vi "Initialize.vi"(8 "error in":errorcluster, 11 "Plugin in":refnum<class "Sequencer with Output Values.lvclass">) -> (0 "error out":errorcluster, 3 "Plugin out":refnum<class "Sequencer with Output Values.lvclass">)   [LabVIEW 2024, in "Sequencer with Output Values.lvlib" / "Sequencer with Output Values.lvclass"]
uses:
  Sequencer with Output Values.lvclass
  C:/Program Files/National Instruments/LabVIEW 2024/vi.lib/FlexLogger/SDK/PluginSDK.lvlibp/PEFClasses/SDK/Plugin/Plugin.lvclass
  <vilib>/FlexLogger/SDK/PluginSDK.lvlibp/PEFClasses/SDK/Processing Element/Timing Parameters.ctl
  <vilib>/FlexLogger/SDK/PluginSDK.lvlibp/PEFClasses/SDK/Processing Element/Timing Method.ctl
  Params.ctl
  Step Settings.ctl
  Helper VIs/Cust UI.ctl
  Sequencer with Output Values.lvclass/Sequencer with Output Values.ctl
  <vilib>/FlexLogger/SDK/PluginSDK.lvlibp/PEFClasses/SDK/Producer Channel/Producer Channel.lvclass
  C:/Program Files/National Instruments/LabVIEW 2024/vi.lib/FlexLogger/SDK/PluginSDK.lvlibp/PEFClasses/SDK/Channel/Channel.lvclass
  Global Strings.vi
  <vilib>/FlexLogger/SDK/PluginSDK.lvlibp/PEFClasses/SDK/Plugin/ParameterAccess/Write Command.vi
  <vilib>/FlexLogger/SDK/PluginSDK.lvlibp/PEFClasses/SDK/Plugin/ParameterAccess/Read String.vi
  <vilib>/FlexLogger/SDK/PluginSDK.lvlibp/PEFClasses/SDK/Plugin/ParameterAccess/Write String.vi
  Settings UI.vi
  <vilib>/FlexLogger/SDK/PluginSDK.lvlibp/PEFClasses/SDK/Producer Channel/Create Producer Channel.vi
  <vilib>/FlexLogger/SDK/PluginSDK.lvlibp/PEFClasses/SDK/Plugin/Plugin.lvclass
  <vilib>/FlexLogger/SDK/PluginSDK.lvlibp/PEFClasses/SDK/Processing Element/Processing Element.lvclass
  <vilib>/FlexLogger/SDK/PluginSDK.lvlibp
  C:/Program Files/National Instruments/LabVIEW 2024/vi.lib/FlexLogger/SDK/PluginSDK.lvlibp/PEFClasses/SDK/Processing Element/Processing Element.lvclass
  C:/dev/niflexlogger-plugins/plugins/Sequencer with Output Values/source/Sequencer with Output Values/Sequencer with Output Values.lvclass
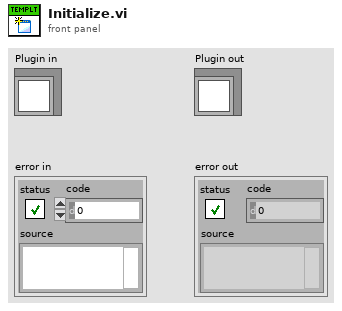
[diagram p1: front panel]
types:
  T1 = typedef "Sequencer with Output Values.lvlib/Sequencer with Output Values.lvclass/Cust UI.ctl" = refnum<vi>
  T2 = typedef "Sequencer with Output Values.lvlib/Sequencer with Output Values.lvclass/Step Settings.ctl" = cluster{"Duration":dbl, "Mode":string, "Delay Between Values":dbl, "Analog Values":string[], "Digital Values":string[]}
  T3 = typedef "Sequencer with Output Values.lvlib/Sequencer with Output Values.lvclass/Params.ctl" = cluster{"Step Values":T2[], "Only Execute When Test Running":bool, "Reset Sequence When Test Starts":bool, "Current Sequence ID":u32, "Total Iterations":u32, "Current Step Start Timestamp":dbl, "Number of Sequence Steps":i32, "Num of Analog Channels":i32, "Num of Digital Channels":i32, "Delay Before Starting Sequence":dbl, "Show UI":bool, "Time Remaining":dbl, "Test Running":bool, "Pause Timestamp":dbl, "Default Analog Values":dbl[], "Default Digital Values":bool[]}
  T4 = typedef "PluginSDK.lvlibp/Processing Element.lvclass/Timing Parameters.ctl" = cluster{"Timing Method":T5, "Timing Period (ms)":i32}
  T5 = typedef "PluginSDK.lvlibp/Processing Element.lvclass/Timing Method.ctl" = enum16{"Periodic", "Immediate", "On Data Ready", "Triggered"}
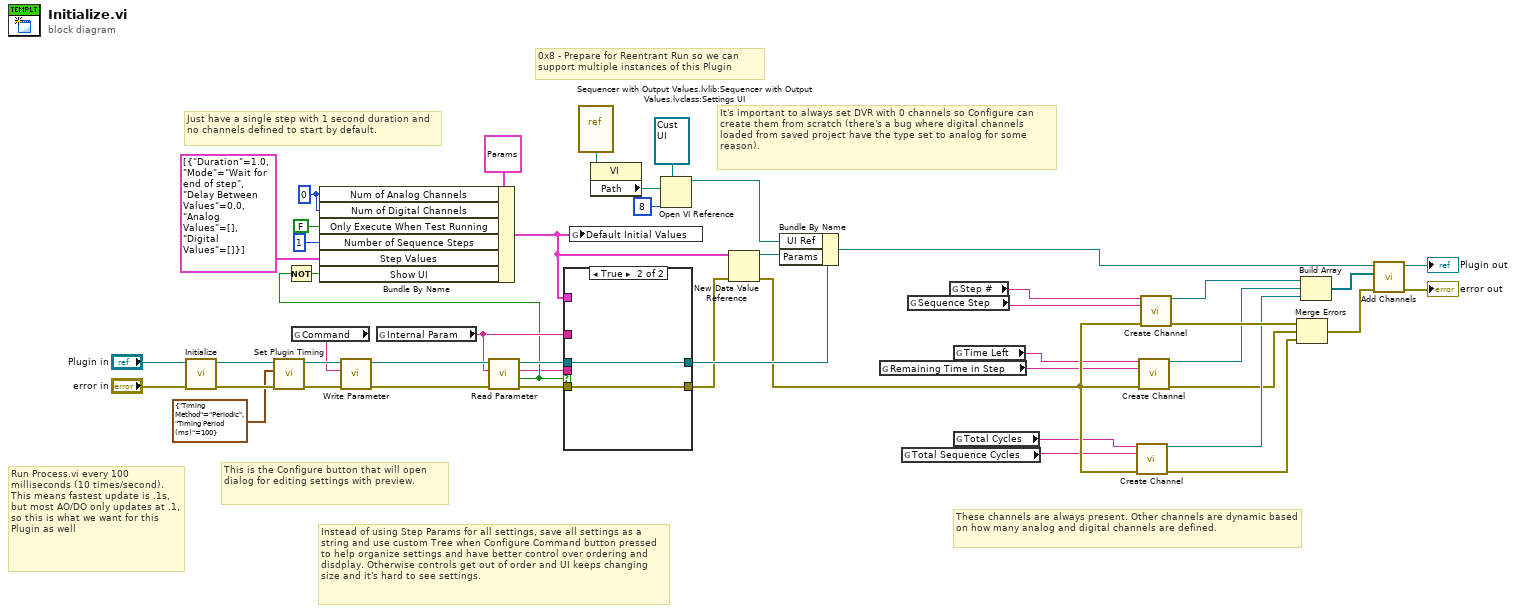
[diagram p0: block diagram]
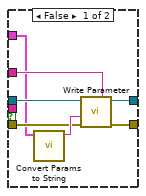
[diagram p2: hidden frame]
diagram:
  w21 = 0 ("Num of Analog Channels")
  # "0x8 - Prepare for Reentrant Run so we can support multiple instances of this Plugin"
  # "It's important to always set DVR with 0 channels so Configure can create them from scratch (there's a bug where digital channels loaded from saved project have the type set to analog for some reason)."
  # "This is the Configure button that will open dialog for editing settings with preview."
  # "Instead of using Step Params for all settings, save all settings as a string and use custom Tree when Configure Command button pressed to help organize settings and have better control over ordering and disdplay. Otherwise controls get out of order and UI keeps changing size and it's hard to see settings."
  # "Just have a single step with 1 second duration and no channels defined to start by default."
  # "These channels are always present. Other channels are dynamic based on how many analog and digital channels are defined."
  # "Run Process.vi every 100 milliseconds (10 times/second). This means fastest update is .1s, but most AO/DO only updates at .1, so this is what we want for this Plugin as well"
  n1 = call-parent "Initialize.vi"("error in (no error)"="error in", "Plugin in"="Plugin in") -> ("error out"=w47:errorcluster, "Plugin out"=w45:refnum<class "Sequencer with Output Values.lvclass">)  [unwired: 8 in]
  n2 = call <vilib>:"Set Plugin Timing.vi"("error in (no error)"=w47, "Timing Parameters"=T4 {"Timing Method"=enum."Periodic", "Timing Period (ms)"=100}, "Plugin in"=w45) -> ("error out"=w31:errorcluster, "Plugin out"=w32:refnum<class "Sequencer with Output Values.lvclass">)  [unwired: 7 in]
  n3 = global read "Global Strings.vi" "Command"() -> (w30:string)
  n4 = call-poly <vilib>:"Write Parameter.vi"("error in (no error)"=w31, "Name"=w30, "Plugin in"=w32) -> ("error out"=w25:errorcluster, "Plugin out"=w26:refnum<class "Sequencer with Output Values.lvclass">)  [unwired: 7 in]
  n5 = global read "Global Strings.vi" "Internal Param"() -> (w22:string)
  n6 = call-poly <vilib>:"Read Parameter.vi"("error in (no error)"=w25, "Name"=w22, "Plugin in"=w26) -> ("error out"=w23:errorcluster, "Found"=w11:bool, "Value"=w10:string, "Plugin out"=w24:refnum<class "Sequencer with Output Values.lvclass">)  [unwired: 5 in]
  n7 = Not(x=w11) -> (.not. x?=w14:bool)
  n8 = Bundle By Name(cluster=T3 {"Step Values"=[], "Only Execute When Test Running"=FALSE, "Reset Sequence When Test Starts"=TRUE, "Current Sequence ID"=0, "Total Iterations"=0, "Current Step Start Timestamp"=-1.0, "Number of Sequence Steps"=0, "Num of Analog Channels"=0, "Num of Digital Channels"=0, "Delay Before Starting Sequence"=0.0, "Show UI"=FALSE, "Time Remaining"=0.0, "Test Running"=FALSE, "Pause Timestamp"=0.0, "Default Analog Values"=[], "Default Digital Values"=[]}, "Num of Analog Channels"=w21, "Num of Digital Channels"=w21, "Only Execute When Test Running"=FALSE, "Number of Sequence Steps"=1, "Step Values"=T2[] [{"Duration"=1.0, "Mode"="Wait for end of step", "Delay Between Values"=0.0, "Analog Values"=[], "Digital Values"=[]}], "Show UI"=w14) -> (w15:T3)
  n9 = case shown="True" w11 {
    tunnel: w15 -> [w49 _]
    tunnel: [w54 w56] -> w17
    tunnel: [w53 w57] -> w28
    tunnel: w24 -> [w52 w57]
    tunnel: w23 -> [w51 w56]
    tunnel: w22 -> [w50 _]
    tunnel: w10 -> [_ _]
    frame False {
      n10 = call "Convert Params to String.vi"("Settings"=w49) -> ("String out"=w55:string)  [unwired: 10 in]
      n11 = call-poly <vilib>:"Write Parameter.vi"("error in (no error)"=w51, "Value"=w55, "Name"=w50, "Plugin in"=w52) -> ("error out"=w54:errorcluster, "Plugin out"=w53:refnum<class "Sequencer with Output Values.lvclass">)  [unwired: 6 in]
    }
    frame True {
    }
  }
  n12 = global write "Global Strings.vi" "Default Initial Values"(w15) -> ()
  n13 = vi-ref "Sequencer with Output Values.lvlib:Sequencer with Output Values.lvclass:Settings UI.vi"() -> (w13:refnum<vi>)
  n14 = property class="VI"(reference=w13) -> ("Path"=w20:path)  [unwired: 1 in, 2 out]
  n15 = Open VI Reference(type specifier VI Refnum (for type only)=T1 refnum ("Cust UI"), vi path=w20, options=8) -> (vi reference=w12:T1)  [unwired: 3 in, 1 out]
  n16 = New Data Value Reference(data value=w15, error in=w17) -> (data value reference=w19:refnum<data-value>, error out=w16:errorcluster)
  n17 = Bundle By Name(cluster=w28, "UI Ref"=w12, "Params"=w19) -> (w27:refnum<class "Sequencer with Output Values.lvclass">)
  n18 = global read "Global Strings.vi" "Remaining Time in Step"() -> (w4:string)
  n19 = global read "Global Strings.vi" "Total Sequence Cycles"() -> (w2:string)
  n20 = global read "Global Strings.vi" "Sequence Step"() -> (w6:string)
  n21 = global read "Global Strings.vi" "Step #"() -> (w5:string)
  n22 = global read "Global Strings.vi" "Time Left"() -> (w3:string)
  n23 = global read "Global Strings.vi" "Total Cycles"() -> (w1:string)
  n24 = call-poly <vilib>:"Create Channel.vi"("Unique Channel Identifier"=w1, "Default Channel Name"=w2, "error in (no error)"=w16) -> ("Producer Channel"=w38:refnum<class "Producer Channel.lvclass">, "error out"=w36:errorcluster)  [unwired: 11 in]
  n25 = call-poly <vilib>:"Create Channel.vi"("Unique Channel Identifier"=w3, "Default Channel Name"=w4, "error in (no error)"=w16) -> ("Producer Channel"=w39:refnum<class "Producer Channel.lvclass">, "error out"=w37:errorcluster)  [unwired: 11 in]
  n26 = call-poly <vilib>:"Create Channel.vi"("Unique Channel Identifier"=w5, "Default Channel Name"=w6, "error in (no error)"=w16) -> ("Producer Channel"=w40:refnum<class "Producer Channel.lvclass">, "error out"=w41:errorcluster)  [unwired: 11 in]
  n27 = Merge Errors(w41, w37, w36) -> (w43:errorcluster)
  n28 = Build Array(w40, w39, w38) -> (w44:refnum<class "Producer Channel.lvclass">[])
  n29 = call <vilib>:"Add Channels.vi"("error in (no error)"=w43, "Channels"=w44, "Plugin in"=w27) -> ("error out"=→"error out":errorcluster, "Plugin out"=→"Plugin out":refnum<class "Sequencer with Output Values.lvclass">)  [unwired: 7 in]
